vi "Add Item to Menu.vi"(5 "Create Submenu if a Cluster":bool, 6 "tag prefix":string, 7 "menu tag":string, 8 "error in (no error)":errorcluster, 9 "after item":string caption="after item (Default=end; '-1'=start)", 10 "Item(s) to Add":variant, 11 "menu reference":refnum<k9>) -> (0 "error out":errorcluster, 1 "last root-level item":string, 3 "menu reference out":refnum<k9>)   [LabVIEW 2019, in "Menu From Cluster.lvlib"]
doc: "Use an input value to set menu items. The input value can be an enum or a boolean, or a cluster of such types. \n\n'After item' can be the tag of an item, or empty to menn insert at end, or \"-1\" to insert at front."
uses:
  Menu From Cluster.lvlib
  <vilib>/Utility/VariantDataType/VariantType.lvlib
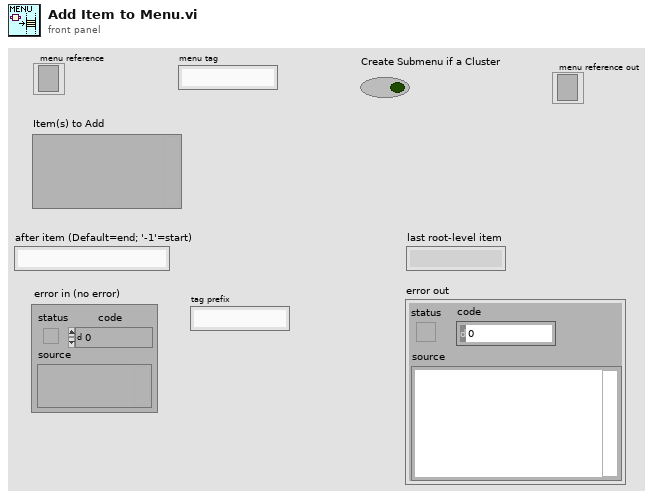
[diagram p1: front panel]
types:
  T1 = typedef "VariantType.lvlib/Type.ctl" = enum8{"Invalid Type", "Void", "I8", "I16", "I32", "I64", "U8", "U16", "U32", "U64", "Single Float", "Double Float", "Extended Float", "Single Complex", "Double Complex", "Extended Complex", "Enum U8", "Enum U16", "Enum U32", "Enum U64", "Single Float With Unit", "Double Float With Unit", "Extended Float With Unit", "Single Complex with Unit", "Double Complex with Unit", "Extended Complex with Unit", "Boolean", "String", "Path", "Picture", "Tag", "Array", "Cluster", "Variant", "LV Variant", "Waveform", "Timestamp", "Digital Waveform", "Digital Data", "ExpressData", "Refnum", "External Data", "VI", "Poly VI", "LabVIEW Class Instance", "Fixed Point"}
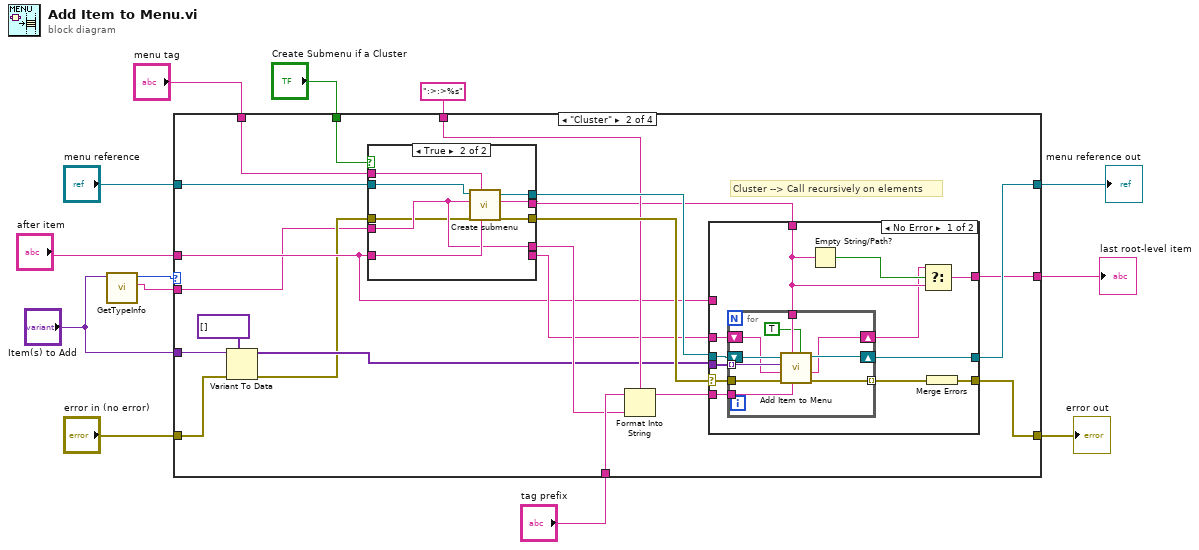
[diagram p0: block diagram]
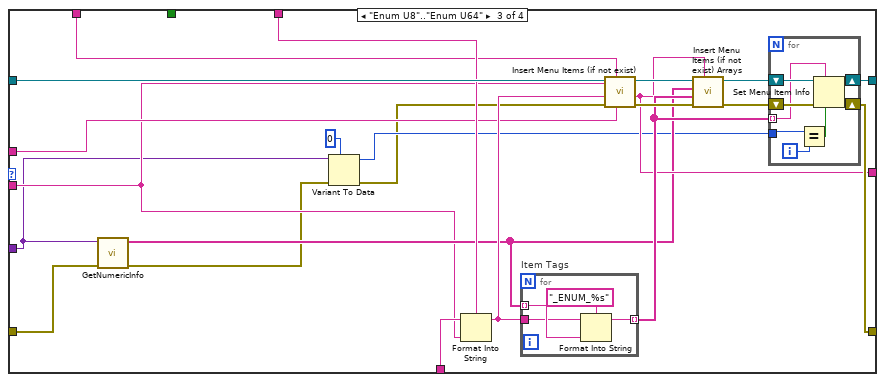
[diagram p5: hidden frame]
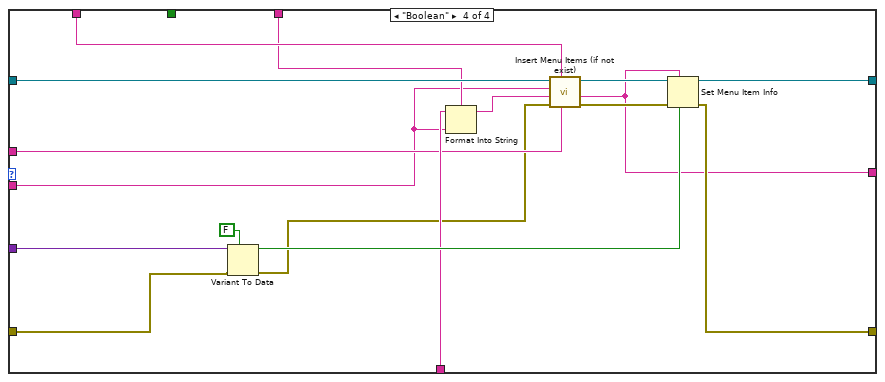
[diagram p6: hidden frame]
diagram:
  n1 = call <vilib>:"GetTypeInfo.vi"("Variant"="Item(s) to Add") -> ("Name"=w1:string, "Type Enum"=w3:T1)  [unwired: 6 in, 3 out]
  n2 = case shown="\"Cluster\"" w3 {
    tunnel: "menu reference" -> [w15 w35 w92 w123]
    tunnel: "error in (no error)" -> [w16 w19 w76 w109]
    tunnel: [w16 w37 w91 w119] -> w11
    tunnel: "menu tag" -> [_ w33 w87 w120]
    tunnel: [w15 w36 w90 w118] -> w9
    tunnel: "Create Submenu if a Cluster" -> [_ w32 _ _]
    tunnel: "tag prefix" -> [_ w30 w89 w116]
    tunnel: ":>:>%s" ("format string") -> [_ w29 w88 w115]
    tunnel: "after item" -> [w14 w23 w84 w114]
    tunnel: [w14 w24 w83 w113] -> w4
    tunnel: "Item(s) to Add" -> [_ w22 w79 w110]
    tunnel: w1 -> [_ w17 w81 w112]
    frame "Invalid Type", Default {
    }
    frame "Cluster" {
      # "Cluster --> Call recursively on elements"
      n3 = Variant To Data(error in=w19, type=variant[] [], Variant=w22) -> (data=w20:variant[], error out=w18:errorcluster)
      n4 = case shown="True" w32 {
        tunnel: w35 -> [w40 w46]
        tunnel: [w40 w49] -> w34
        tunnel: w33 -> [w39 w45]
        tunnel: [w39 w48] -> w28
        tunnel: [w41 w47] -> w31
        tunnel: w18 -> [w41 w42]
        tunnel: [_ w43] -> w26
        tunnel: w23 -> [w38 w44]
        tunnel: [w38 _] -> w25
        tunnel: w17 -> [_ w43]
        frame False {
        }
        frame True {
          n5 = call "Create submenu.vi"("after item"=w44, "owning menu tag"=w45, "error in (no error)"=w42, "tag in"=w43, "Menu in"=w46) -> ("error out"=w47:errorcluster, "tag out"=w48:string, "Menu out"=w49:refnum<k9>)  [unwired: 4 in]
        }
      }
      n6 = Format Into String(format string=w29, initial string=w30, w26) -> (resulting string=w27:string)  [unwired: 1 in, 1 out]
      n7 = case shown="No Error" w31 {
        selector: w31 -> [w59 w74]
        tunnel: w20 -> [w61 _]
        tunnel: w34 -> [w60 w73]
        tunnel: [w57 w74] -> w37
        tunnel: w28 -> [w52 _]
        tunnel: [w56 w73] -> w36
        tunnel: w27 -> [w55 _]
        tunnel: w25 -> [w54 _]
        tunnel: [w51 w72] -> w24
        tunnel: w23 -> [_ w72]
        frame No Error {
          n8 = for {
            tunnel: w61 -> [w70] mode=indexing
            tunnel: w59 -> [w69]
            tunnel: [w68] -> w58 mode=indexing
            tunnel: w52 -> [w67]
            shift-right: [w66] -> w56
            shift-left: w60 -> [w71]
            tunnel: w55 -> [w65]
            shift-right: [w62] -> w50
            shift-left: w54 -> [w63]
            n9 = call "Add Item to Menu.vi"("Create Submenu if a Cluster"=TRUE, "tag prefix"=w65, "menu tag"=w67, "error in (no error)"=w69, "after item"=w63, "Item(s) to Add"=w70, "menu reference"=w71) -> ("error out"=w68:errorcluster, "last root-level item"=w62:string, "menu reference out"=w66:refnum<k9>)  [unwired: 2 in]
          }
          n10 = Empty String/Path?(string/path=w52) -> (empty?=w53:bool)
          n11 = Select(t=w50, s=w53, f=w52) -> (s? t:f=w51:string)
          n12 = Merge Errors(w58) -> (w57:errorcluster)
        }
        frame Error {
        }
      }
    }
    frame "Enum U8".."Enum U64" {
      n13 = call <vilib>:"GetNumericInfo.vi"("error in (no error)"=w76, "Variant"=w79) -> ("error out"=w77:errorcluster, "EnumNames"=w82:string[])  [unwired: 6 in, 2 out]
      n14 = Variant To Data(error in=w77, type=u64 0, Variant=w79) -> (data=w78:u64, error out=w75:errorcluster)
      n15 = Format Into String(format string=w88, initial string=w89, w81) -> (resulting string=w86:string)  [unwired: 1 in, 1 out]
      n16 = for "Item Tags" {
        tunnel: w86 -> [w107]
        tunnel: w82 -> [w108] mode=indexing
        tunnel: [w105] -> w85 mode=indexing
        n17 = Format Into String(format string="_ENUM_%s", initial string=w107, w108) -> (resulting string=w105:string)  [unwired: 1 in, 1 out]
      }
      n18 = call "Insert Menu Items (if not exist).vi"("after item"=w84, "menu tag"=w87, "error in (no error)"=w75, "item tag"=w86, "item name"=w81, "Menu in"=w92) -> ("error out"=w96:errorcluster, "tag out"=w83:string, "Menu out"=w95:refnum<k9>)  [unwired: 3 in]
      n19 = call "Insert Menu Items (if not exist) Arrays.vi"("menu tag"=w83, "error in (no error)"=w96, "Item tags"=w85, "Item names"=w82, "Menu in"=w95) -> ("error out"=w94:errorcluster, "Menu out"=w93:refnum<k9>)  [unwired: 5 in]
      n20 = for {
        shift-right: [w101] -> w90
        shift-left: w93 -> [w103]
        shift-right: [w102] -> w91
        shift-left: w94 -> [w104]
        tunnel: w85 -> [w100] mode=indexing
        tunnel: w78 -> [w98]
        i -> [w99]
        n21 = Equal?(x=w98, y=w99) -> (x = y?=w97:bool)
        n22 = Set Menu Item Info(6:w97, 7:w100, 8:w104, 11:w103) -> (0:w102:errorcluster, 3:w101:refnum<k9>)  [unwired: 3 out]
      }
    }
    frame "Boolean" {
      n23 = Variant To Data(error in=w109, type=FALSE, Variant=w110) -> (data=w121:bool, error out=w111:errorcluster)
      n24 = Format Into String(format string=w115, initial string=w116, w112) -> (resulting string=w117:string)  [unwired: 1 in, 1 out]
      n25 = call "Insert Menu Items (if not exist).vi"("after item"=w114, "menu tag"=w120, "error in (no error)"=w111, "item tag"=w117, "item name"=w112, "Menu in"=w123) -> ("error out"=w125:errorcluster, "tag out"=w113:string, "Menu out"=w124:refnum<k9>)  [unwired: 3 in]
      n26 = Set Menu Item Info(6:w121, 7:w113, 8:w125, 11:w124) -> (0:w119:errorcluster, 3:w118:refnum<k9>)  [unwired: 3 out]
    }
  }
  "error out" <- w11
  "menu reference out" <- w9
  "last root-level item" <- w4
